vi "SPI Write Read 1 Frame.vi"(5 "CS Configuration":T1={"CS Channel"=7, "CS Logic Level"=enum."Active High"}, 7 "SPI Channel (0)":u8, 8 "Error In":errorcluster, 10 "Data":u8[](array[numeric]), 11 "LINX Resource":T3={"IO"=enum."Remote", "Interface"=enum."TCP", "LINX Device Config"={"Interface"=enum."TCP", "COM Port"="N/A", "TCP Configuration"={"IP Address"="raspberrypi", "Port"=44301}, "Device Family"=4, "Device ID"=3, "Device Name"="Raspberry Pi 2 Model B\u0000", "TCP Ref"=refnum, "Channels"={"DI"=[7, 11, 12, 13, 15, 16, 18, 22, 29, 31, 32, 33, 35, 36, 37, 38, 40], "DO"=[7, 11, 12, 13, 15, 16, 18, 22, 29, 31, 32, 33, 35, 36, 37, 38, 40], "AI"=[], "AO"=[], "PWM"=[], "QE"=[], "UART"=[0], "I2C 2"=[1], "SPI"=[0], "CAN"=[], "Servo"=[], "AI Ref (V)"=0.0, "AI Resolution (Bits)"=0, "AO Ref (V)"=0.0, "AO Resolution (Bits)"=0}}}) -> (0 "Error Out":errorcluster, 2 "Read Data":u8[](array[numeric]), 3 "LINX Resource":T3={"IO"=enum."Remote", "Interface"=enum."TCP", "LINX Device Config"={"Interface"=enum."TCP", "COM Port"="N/A", "TCP Configuration"={"IP Address"="raspberrypi", "Port"=44301}, "Device Family"=4, "Device ID"=3, "Device Name"="Raspberry Pi 2 Model B\u0000", "TCP Ref"=refnum, "Channels"={"DI"=[7, 11, 12, 13, 15, 16, 18, 22, 29, 31, 32, 33, 35, 36, 37, 38, 40], "DO"=[7, 11, 12, 13, 15, 16, 18, 22, 29, 31, 32, 33, 35, 36, 37, 38, 40], "AI"=[], "AO"=[], "PWM"=[], "QE"=[], "UART"=[0], "I2C 2"=[1], "SPI"=[0], "CAN"=[], "Servo"=[], "AI Ref (V)"=0.0, "AI Resolution (Bits)"=0, "AO Ref (V)"=0.0, "AO Resolution (Bits)"=0}}}, 4 "status":i32)   [LabVIEW 2014, in "LMH-LINX.lvlib"]
doc: "Transmit data on the specified SPI channel and read the response. This VI transmits the entire data input in a single frame by setting CS active, shifting out all bytes in data, then setting CS idle.\n\nSPI is full duplex, therefore the write and read operations take place simultaneously.\n\n<b>SPI Channel</b> specifies the SPI channel to write/read to.\n\n<b>Data</b> is a U8 array of data bytes to shift out starting with Data[0] to Data[n-1].\n\n<b>CS Channel</b> specifies the Chip Select (DIO) channel to use during the SPI transaction.\n\n<b>CS Logic Level</b> specifies the polarity of the chip select output. Active low is most common and results in CS starting in the idle/high state and data being trasnmitted after CS is driven to the active/low state."
uses:
  LMH-LINX.lvlib
  Private/Type Defs/LINX Ref.ctl
  Private/Type Defs/Platform.ctl
  Private/Type Defs/Interface.ctl
  Private/Device/Type Defs/LINX Device Config.ctl
  Private/Device/Type Defs/TCP Config.ctl
  Private/Device/Type Defs/Channels.ctl
  SPI CS Config.ctl
  Private/Type Defs/Peripherals/SPI/SPI CS Logic Level.ctl
  Private/Local IO/LinxSpiWriteRead.vi
  Utilities/Check Channel.vi
  Private/Utilties/Generate Error.vi
  Private/Device/Peripheral/SPI/SPI Write Read.vi
  Private/Device/Device.lvlib
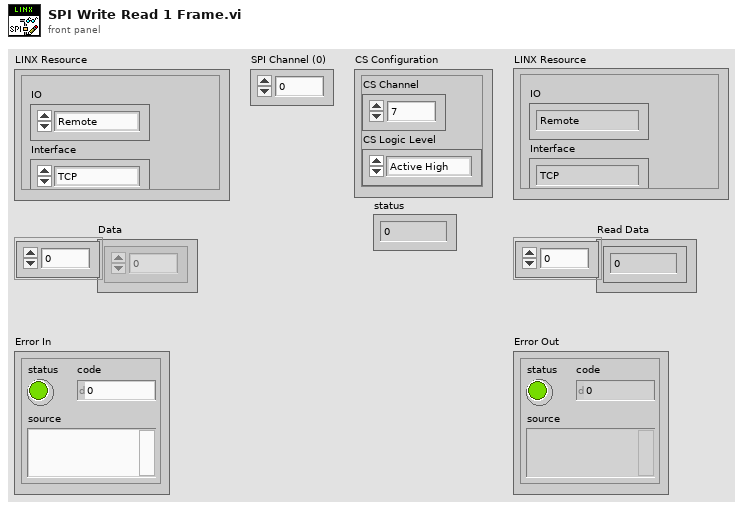
[diagram p1: front panel]
types:
  T1 = typedef "LMH-LINX.lvlib/SPI CS Config.ctl" = cluster{"CS Channel":u8, "CS Logic Level":T2}
  T2 = typedef "LMH-LINX.lvlib/SPI CS Logic Level.ctl" = enum8{"Active Low", "Active High"}
  T3 = typedef "LMH-LINX.lvlib/LINX Ref.ctl" = cluster{"IO":T4, "Interface":T5, "LINX Device Config":T6}
  T4 = typedef "LMH-LINX.lvlib/Platform.ctl" = enum16{"Remote", "Local"}
  T5 = typedef "LMH-LINX.lvlib/Interface.ctl" = enum16{"Serial", "TCP"}
  T6 = typedef "LMH-LINX.lvlib/Device.lvlib/LINX Device Config.ctl" = cluster{"Interface":T5, "COM Port":refnum<visa-resource-name>, "TCP Configuration":T7, "Device Family":u8, "Device ID":u8, "Device Name":string, "TCP Ref":refnum<k5>, "Channels":T8}
  T7 = typedef "LMH-LINX.lvlib/Device.lvlib/TCP Config.ctl" = cluster{"IP Address":string, "Port":u16}
  T8 = typedef "LMH-LINX.lvlib/Channels.ctl" = cluster{"DI":u8[], "DO":u8[], "AI":u8[], "AO":u8[], "PWM":u8[], "QE":u8[], "UART":u8[], "I2C 2":u8[], "SPI":u8[], "CAN":u8[], "Servo":u8[], "AI Ref (V)":dbl, "AI Resolution (Bits)":u8, "AO Ref (V)":dbl, "AO Resolution (Bits)":u8}
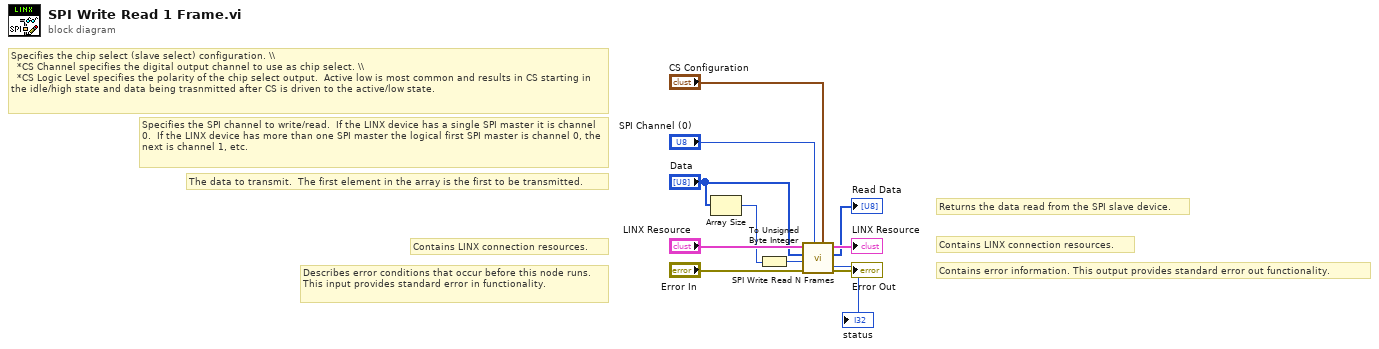
[diagram p0: block diagram]
diagram:
  # "The data to transmit.  The first element in the array is the first to be transmitted."
  # "Specifies the SPI channel to write/read.  If the LINX device has a single SPI master it is channel 0.  If the LINX device has more than one SPI master the logical first SPI master is channel 0, the next is channel 1, etc."
  # "Specifies the chip select (slave select) configuration. \\\\\n  *CS Channel specifies the digital output channel to use as chip select. \\\\ \n  *CS Logic Level specifies the polarity of the chip select output.  Active low is most common and results in CS starting in the idle/high state and data being trasnmitted after CS is driven to the active/low state."
  # "Returns the data read from the SPI slave device."
  # "Contains LINX connection resources."
  # "Contains error information. This output provides standard error out functionality."
  # "Contains LINX connection resources."
  # "Describes error conditions that occur before this node runs. This input provides standard error in functionality."
  n1 = Array Size(array="Data") -> (size(s)=w4:i32)
  n2 = To Unsigned Byte Integer(number=w4) -> (unsigned 8bit integer=w3:u8)
  n3 = call "SPI Write Read N Frames.vi"("CS Configuration"="CS Configuration", "SPI Channel (0)"="SPI Channel (0)", "Error In"="Error In", "SPI Frame Size"=w3, "Data"="Data", "LINX Resource"="LINX Resource") -> ("Error Out"=→"Error Out":errorcluster, "Read Data"=→"Read Data":u8[], "LINX Resource"=→"LINX Resource":T3, "status"=→"status":i32)  [unwired: 2 in]
